vi "Create Map from Messages to Value Indexes.vi"(10 "1553 channel handles":T1[](array[typedef]) {"messages"."Rx status handles" format="%.0x"; "messages"."Tx status handles" format="%.0x"; "messages"."timestamps" format="%.0x"; "messages"."parameters"."RxBC channel handle" format="%.0x"; "messages"."parameters"."RxRT channel handle" format="%.0x"; "messages"."parameters"."Tx channel handle" format="%.0x"}, 11 "1553 channels":T5[](array[typedef])) -> (3 "map from messages to value indexes":T11)   [LabVIEW 2020, in "Ballard MIL-STD-1553 Engine.lvlib" / "Custom Device.lvlib"]
uses:
  Custom Device.lvlib
  Shared/Map of Messages to Value Indexes.ctl
  Shared/Message Map Key.ctl
  Implementation/Rx Execution Unit/Message Map Value.ctl
  Shared/Message Definition.ctl
  Shared/Message Type.ctl
  Shared/Terminal Endpoint.ctl
  Shared/Address.ctl
  Shared/Parameter Definition.ctl
  Shared/1553 Channel.ctl
  Implementation/Execution Unit/1553 Channel Handles.ctl
  Implementation/Execution Unit/Message Handles.ctl
  Implementation/Execution Unit/Parameter Handles.ctl
  <vilib>/NI VeriStand/Custom Device API/Custom Device Item Ref.ctl
  Implementation/Rx Execution Unit/Rx Execution Unit.lvclass
  <vilib>/NI VeriStand/Custom Device API/Custom Device API.lvlib
  Implementation/Execution Unit/Execution Unit.lvclass
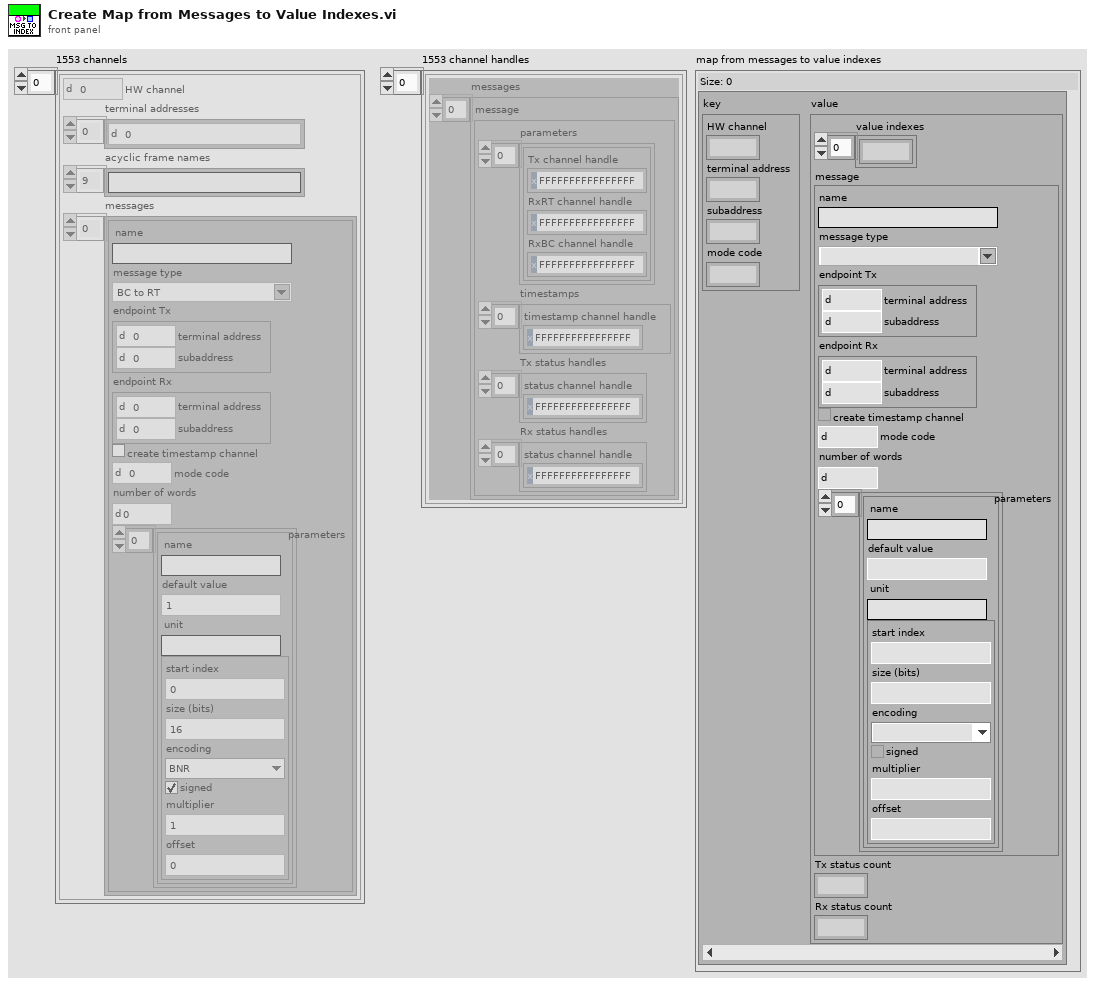
[diagram p1: front panel]
types:
  T1 = typedef "Ballard MIL-STD-1553 Engine.lvlib/Implementation.lvlib/Execution Unit.lvclass/1553 Channel Handles.ctl" = cluster{"messages":T2[]}
  T2 = typedef "Ballard MIL-STD-1553 Engine.lvlib/Implementation.lvlib/Execution Unit.lvclass/Message Handles.ctl" = cluster{"parameters":T3[], "timestamps":T4[], "Tx status handles":T4[], "Rx status handles":T4[]}
  T3 = typedef "Ballard MIL-STD-1553 Engine.lvlib/Implementation.lvlib/Execution Unit.lvclass/Parameter Handles.ctl" = cluster{"Tx channel handle":T4, "RxRT channel handle":T4, "RxBC channel handle":T4}
  T4 = typedef "Custom Device API.lvlib/Custom Device Item Ref.ctl" = u64
  T5 = typedef "1553 Channel.ctl" = cluster{"HW channel":u16, "terminal addresses":T6[], "acyclic frame names":string[], "messages":T7[]}
  T6 = typedef "Address.ctl" = u16
  T7 = typedef "Message Definition.ctl" = cluster{"name":string, "message type":T8, "endpoint Tx":T9, "endpoint Rx":T9, "create timestamp channel":bool, "mode code":u16, "number of words":u16, "parameters":cluster{"name":string, "default value":dbl, "unit":string, "parameter definition":T10}[]}
  T8 = typedef "Message Type.ctl" = string
  T9 = typedef "Terminal Endpoint.ctl" = cluster{"terminal address":T6, "subaddress":T6}
  T10 = typedef "Parameter Definition.ctl" = cluster{"start index":i32, "size (bits)":i32, "encoding":enum16{"BNR", "BCD", "Discrete"}, "signed":bool, "multiplier":dbl, "offset":dbl}
  T11 = typedef "Map of Messages to Value Indexes.ctl" = map{T12, T13}
  T12 = typedef "Message Map Key.ctl" = cluster{"HW channel":u16, "terminal address":u16, "subaddress":u16, "mode code":u16}
  T13 = typedef "Ballard MIL-STD-1553 Engine.lvlib/Implementation.lvlib/Rx Execution Unit.lvclass/Message Map Value.ctl" = cluster{"value indexes":i32[], "message":T7, "Tx status count":i32, "Rx status count":i32}
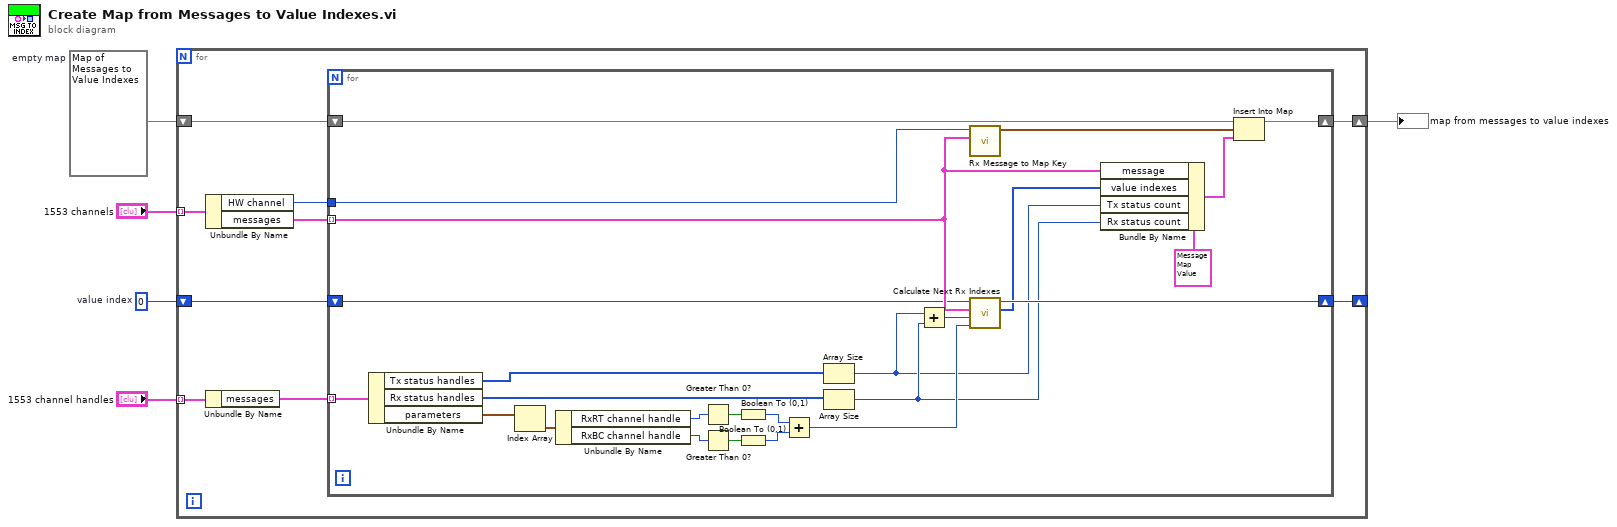
[diagram p0: block diagram]
diagram:
  w3 = 0  # value index
  w5 = T11 {}  # empty map
  n1 = for {
    tunnel: "1553 channels" -> [w14] mode=indexing
    shift-right: [w8] -> w1
    shift-left: w5 -> [w13]
    shift-right: [w9] -> _
    shift-left: w3 -> [w10]
    tunnel: "1553 channel handles" -> [w7] mode=indexing
    n2 = Unbundle By Name(w14) -> ("HW channel"=w12:u16, "messages"=w11:T7[])
    n3 = Unbundle By Name(w7) -> ("messages"=w6:T2[])
    n4 = for {
      tunnel: w12 -> [w37]
      tunnel: w11 -> [w35] mode=indexing
      shift-right: [w39] -> w8
      shift-left: w13 -> [w38]
      shift-right: [w36] -> w9
      shift-left: w10 -> [w34]
      tunnel: w6 -> [w33] mode=indexing
      n5 = Unbundle By Name(w33) -> ("Tx status handles"=w21:T4[], "Rx status handles"=w23:T4[], "parameters"=w32:T3[])
      n6 = Index Array(array=w32) -> (element=w31:T3)  [unwired: 1 in]
      n7 = Unbundle By Name(w31) -> ("RxRT channel handle"=w29:T4, "RxBC channel handle"=w30:T4)
      n8 = Greater Than 0?(x=w29) -> (x > 0?=w27:bool)
      n9 = Greater Than 0?(x=w30) -> (x > 0?=w28:bool)
      n10 = Boolean To (0,1)(Boolean=w27) -> (0, 1=w26:i16)
      n11 = Boolean To (0,1)(Boolean=w28) -> (0, 1=w25:i16)
      n12 = Add(x=w26, y=w25) -> (x+y=w24:i16)
      n13 = Array Size(array=w21) -> (size(s)=w20:i32)
      n14 = Array Size(array=w23) -> (size(s)=w22:i32)
      n15 = Add(x=w20, y=w22) -> (x+y=w16:i32)
      n16 = call "Rx Message to Map Key.vi"("message"=w35, "HW channel"=w37) -> ("message map key"=w19:T12)  [unwired: 9 in]
      n17 = call "Calculate Next Rx Indexes.vi"("Rx endpoints count"=w24, "status channel count"=w16, "message"=w35, "index"=w34) -> ("indexes"=w15:i32[], "next index"=w36:i32)  [unwired: 6 in]
      n18 = Bundle By Name(cluster=T13 {"value indexes"=[], "message"={"name"="", "message type"="BC to RT", "endpoint Tx"={"terminal address"=0, "subaddress"=0}, "endpoint Rx"={"terminal address"=0, "subaddress"=0}, "create timestamp channel"=FALSE, "mode code"=0, "number of words"=0, "parameters"=[]}, "Tx status count"=0, "Rx status count"=0} ("value"), "message"=w35, "value indexes"=w15, "Tx status count"=w20, "Rx status count"=w22) -> (w17:T13)
      n19 = Insert Into Map(map in=w38, key=w19, value=w17) -> (map out=w39:T11)  [unwired: 2 out]
    }
  }
  "map from messages to value indexes" <- w1
